vi "Memory.Pointer.Set Allocated.vi"(10 "allocated":bool, 11 "Pointer in":refnum<class "Memory.Pointer.lvclass">) -> (3 "Pointer out":refnum<class "Memory.Pointer.lvclass">)   [LabVIEW 2016, in "Memory.lvlib" / "Memory.Pointer.lvclass"]
uses:
  Memory.Pointer.lvclass
  Memory.Pointer.lvclass/Memory.Pointer.ctl
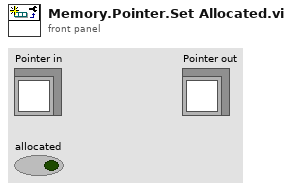
[diagram p1: front panel]
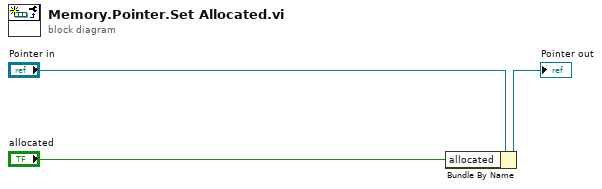
[diagram p0: block diagram]
diagram:
  n1 = Bundle By Name(cluster="Pointer in", "allocated"="allocated") -> (→"Pointer out":refnum<class "Memory.Pointer.lvclass">)
